vi "deleteNot.vi"(8 "error in (no error)":errorcluster, 10 "S/N:":string, 11 "reference in":refnum<class "Notification Controller.lvclass">) -> (0 "error out":errorcluster, 3 "reference out":refnum<class "Notification Controller.lvclass">)   [LabVIEW 2014, in "Notification Controller.lvclass"]
uses:
  Notification Controller.lvclass
  APP/itemsNotification_class/itemsNotification.lvclass
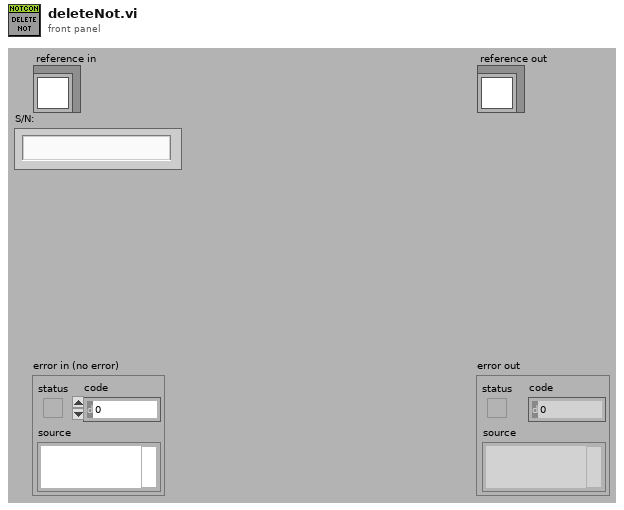
[diagram p1: front panel]
types:
  T1 = typedef "Notification Controller.lvclass/ObjectAttributesRef.ctl" = refnum<data-value>
  T2 = typedef "Notification Controller.lvclass/ObjectAttributes.ctl" = cluster{"MyAttribute":dbl, "items_data":string[][][], "items_notification_refs":refnum<class "itemsNotification.lvclass">[], "notifications_data_items":string[][], "items_nots?":bool, "devices_controller_ref":refnum<class "Devices Controller.lvclass">, "onlineUpdate":timestamp, "notController?":bool, "tracking_notification_ref":refnum<class "trackingNotification.lvclass">, "notifications_data_tracking":string[][], "tracking_parts_data":string[][], "tracking_nots?":bool, "index_tracking_not":i32[], "file_controller_ref":refnum<class "File Controller.lvclass">}
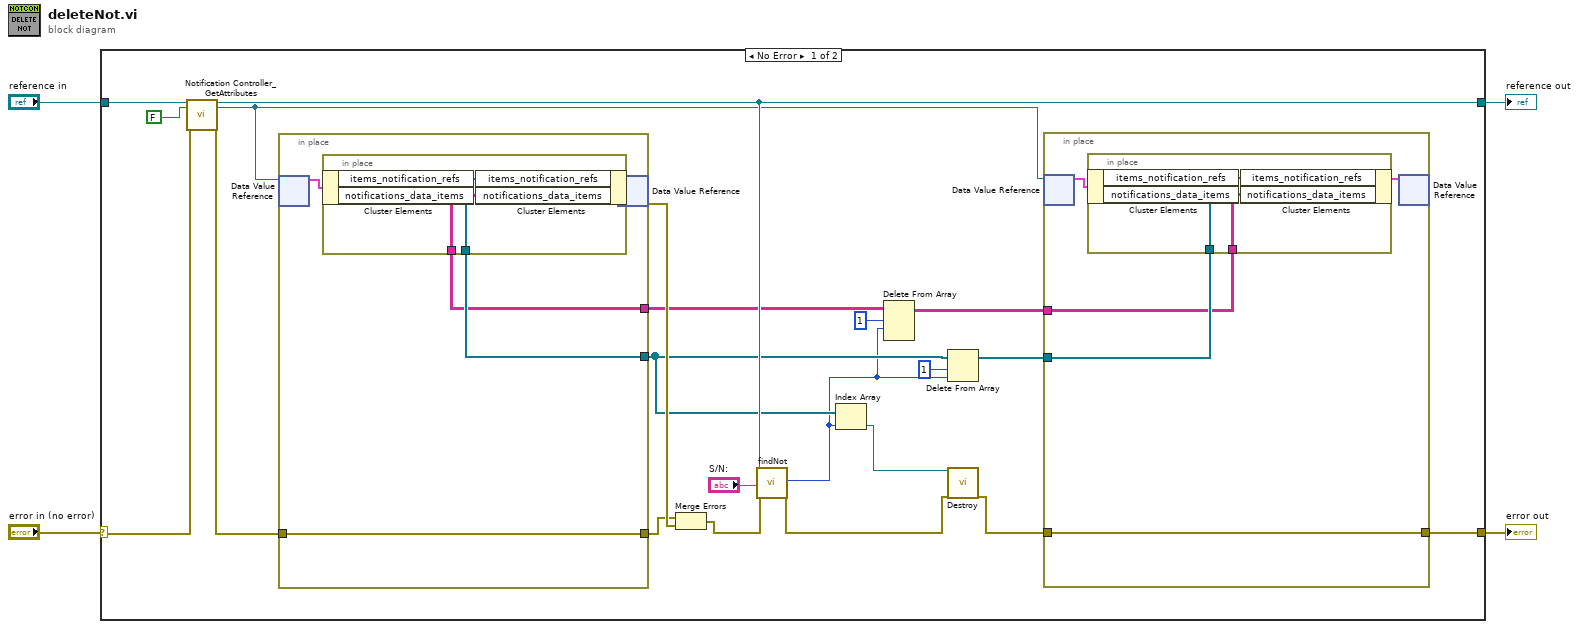
[diagram p0: block diagram]
diagram:
  n1 = case shown="No Error" "error in (no error)" {
    selector: "error in (no error)" -> [w21 w41]
    tunnel: [w13 w41] -> w3
    tunnel: [w19 w40] -> w1
    tunnel: "reference in" -> [w23 w40]
    frame No Error {
      n2 = call "Notification Controller_GetAttributes.vi"("reference in"=w23, "return data? (T)"=FALSE, "error in (no error)"=w21) -> ("reference out"=w19:refnum<class "Notification Controller.lvclass">, "attributes ref"=w12:T1, "error out"=w20:errorcluster)  [unwired: 13 in, 1 out]
      n3 = in-place {
        in-place-border: w20 -> [w35]
        in-place-border: [w35] -> w24
        in-place-border: [w34] -> w11
        in-place-border: [w33] -> w8
        n4 = in-place-dvr #1(w12) -> (w36:T2)  [unwired: 1 out]
        n5 = in-place {
          in-place-border: [w39] -> w34
          in-place-border: [w38] -> w33
          n6 = in-place-cluster #2(w36) -> ("items_notification_refs"=w39:refnum<class "itemsNotification.lvclass">[], "notifications_data_items"=w38:string[][])
          n7 = in-place-cluster #2("items_notification_refs"=w39, "notifications_data_items"=w38) -> (w37:T2)
        }
        n8 = in-place-dvr #1(w37) -> (w25:errorcluster)  [unwired: 1 out]
      }
      n9 = Merge Errors(w24, w25) -> (w18:errorcluster)
      n10 = call "findNot.vi"("reference in"=w19, "S/N:"="S/N:", "error in (no error)"=w18) -> ("index of element"=w5:i32, "error out"=w16:errorcluster)  [unwired: 13 in, 2 out]
      n11 = Index Array(array=w11, index=w5) -> (element=w17:refnum<class "itemsNotification.lvclass">)
      n12 = Delete From Array(array=w8, length=1, index (row)=w5) -> (array with subset deleted=w7:string[][])  [unwired: 1 in, 1 out]
      n13 = Delete From Array(array=w11, length=1, index=w5) -> (array with subset deleted=w9:refnum<class "itemsNotification.lvclass">[])  [unwired: 1 out]
      n14 = call-dynamic "Destroy.vi"("reference in"=w17, "error in (no error)"=w16) -> ("error out"=w14:errorcluster)  [unwired: 16 in, 1 out]
      n15 = in-place {
        in-place-border: w14 -> [w28]
        in-place-border: [w28] -> w13
        in-place-border: w9 -> [w27]
        in-place-border: w7 -> [w26]
        n16 = in-place-dvr #3(w12) -> (w29:T2)  [unwired: 1 out]
        n17 = in-place {
          in-place-border: w27 -> [w32]
          in-place-border: w26 -> [w31]
          n18 = in-place-cluster #4(w29) -> ()  [unwired: 2 out]
          n19 = in-place-cluster #4("items_notification_refs"=w32, "notifications_data_items"=w31) -> (w30:T2)
        }
        n20 = in-place-dvr #3(w30) -> ()  [unwired: 2 out]
      }
    }
    frame Error {
    }
  }
  "error out" <- w3
  "reference out" <- w1
